vi "Initialise.vi"() -> (2 "Pixel Data out":u32[][](array[numeric]), 3 "Scene out":refnum<class "Scene.lvclass">)   [LabVIEW 2022 SP3, in "Benchmark.lvlib"]
uses:
  Benchmark.lvlib
  Main/Scene/Scene.lvclass
  Libraries/Raster/Rectangle Dimensions.ctl
  Libraries/Raster/Raster.lvlib
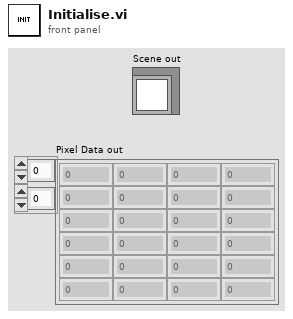
[diagram p1: front panel]
types:
  T1 = typedef "Raster.lvlib/Rectangle Dimensions.ctl" = cluster{"Width":u32, "Height":u32}
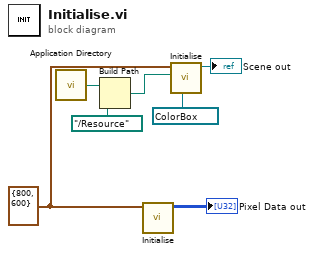
[diagram p0: block diagram]
diagram:
  w7 = T1 {"Width"=800, "Height"=600} ("Screen Dimensions")
  n1 = call <vilib>:"Application Directory.vi"() -> ("Application Directory"=w5:path)
  n2 = Build Path(base path=w5, name or relative path=path "../Resource") -> (appended path=w4:path)
  n3 = call "Initialise.vi"("Screen Dimensions"=w7) -> ("Pixel Data out"=→"Pixel Data out":u32[][])  [unwired: 10 in]
  n4 = call "Initialise.vi"("Diffuse Colour"=refnum<vi> refnum, "Resource Directory"=w4, "Screen Dimensions"=w7) -> ("Scene out"=→"Scene out":refnum<class "Scene.lvclass">)  [unwired: 7 in, 1 out]
